vi "SetProperty.vi"(7 "Property":string, 8 "error in":errorcluster, 10 "Value":string, 11 "camera.nit in":refnum<class "camera.lvclass">) -> (0 "error out":errorcluster)   [LabVIEW 2020, in "camera.lvclass"]
uses:
  camera.lvclass
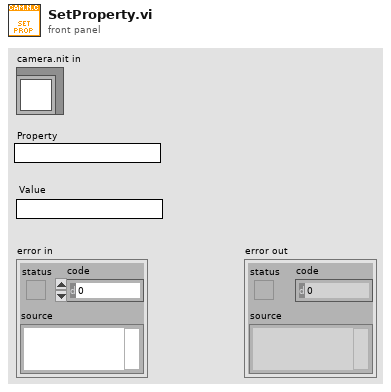
[diagram p1: front panel]
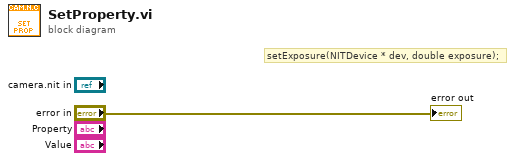
[diagram p0: block diagram]
diagram:
  # "setExposure(NITDevice * dev, double exposure);"
  "error out" <- "error in"
